vi "MGI Origin at Top Left.vi"(7 "Error In":errorcluster, 10 "VI Reference In (Caller)":refnum<vi>) -> (0 "Error Out":errorcluster, 3 "VI Reference Out":refnum<vi>)   [LabVIEW 2016]
doc: "Places the referenced VI's front panel's origin at the top left of the pane.\n\nAuthored by Robert C. Mortensen\nsupport@mooregoodideas.com\nwww.mooregoodideas.com\n\nCopyright (c) 2010, Moore Good Ideas, Inc.\n\nAll rights reserved.\n\nRedistribution and use in source and binary forms, with or without modification, are permitted provided that the following conditions are met:\n\n * Redistributions of source code must retain the above copyright notice, this list of conditions and the following disclaimer.\n * Redistributions in binary form must reproduce the above copyright notice, this list of conditions and the following disclaimer in the documentation and/or other materials provided with the distribution.\n * Neither the name of Moore Good Ideas, Inc. nor the names of its contributors may be used to endorse or promote products derived from this software without specific prior written permission.\n\nTHIS SOFTWARE IS PROVIDED BY THE COPYRIGHT HOLDERS AND CONTRIBUTORS \"AS IS\" AND ANY EXPRESS OR IMPLIED WARRANTIES, INCLUDING, BUT NOT LIMITED TO, THE IMPLIED WARRANTIES OF MERCHANTABILITY AND FITNESS FOR A PARTICULAR PURPOSE ARE DISCLAIMED. IN NO EVENT SHALL THE COPYRIGHT OWNER OR CONTRIBUTORS BE LIABLE FOR ANY DIRECT, INDIRECT, INCIDENTAL, SPECIAL, EXEMPLARY, OR CONSEQUENTIAL DAMAGES (INCLUDING, BUT NOT LIMITED TO, PROCUREMENT OF SUBSTITUTE GOODS OR SERVICES; LOSS OF USE, DATA, OR PROFITS; OR BUSINESS INTERRUPTION) HOWEVER CAUSED AND ON ANY THEORY OF LIABILITY, WHETHER IN CONTRACT, STRICT LIABILITY, OR TORT (INCLUDING NEGLIGENCE OR OTHERWISE) ARISING IN ANY WAY OUT OF THE USE OF THIS SOFTWARE, EVEN IF ADVISED OF THE POSSIBILITY OF SUCH DAMAGE."
uses:
  <vilib>/Utility/miscctls.llb/LVPointTypeDef.ctl
  <userlib>/_MGI/Application Control/MGI VI Reference/MGI Caller's VI Reference.vi
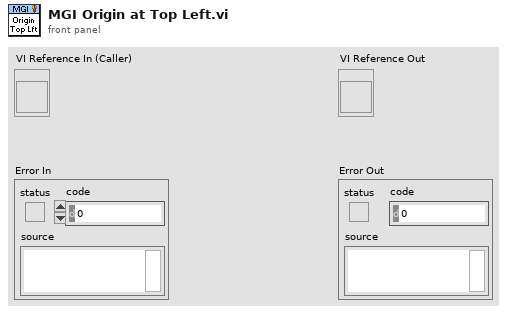
[diagram p1: front panel]
types:
  T1 = typedef "LVPointTypeDef.ctl" = cluster{"Horizontal":i16, "Vertical":i16}
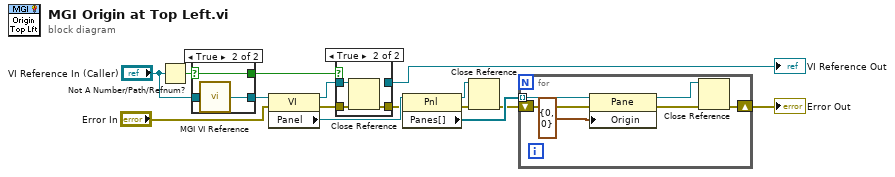
[diagram p0: block diagram]
diagram:
  n1 = Not A Number/Path/Refnum?(number/path/refnum="VI Reference In (Caller)") -> (NaN/Path/Refnum?=w6:bool)
  n2 = case shown="True" w6 {
    selector: w6 -> [_ w17]
    tunnel: [w16 w18] -> w4
    tunnel: "VI Reference In (Caller)" -> [w16 _]
    tunnel: [_ w17] -> w2
    frame False {
    }
    frame True {
      n3 = call-poly <userlib>:"MGI VI Reference.vi"() -> ("Caller's VI Reference"=w18:refnum<vi>)  [unwired: 1 in]
    }
  }
  n4 = property class="VI"(reference=w4, error in="Error In") -> (reference out=w12:refnum<vi>, error out=w13:errorcluster, "Panel"=w15:refnum<vi>)
  n5 = case shown="True" w2 {
    tunnel: w13 -> [w20 w23]
    tunnel: w12 -> [w19 w22]
    tunnel: [w20 w21] -> w11
    tunnel: [w19 _] -> w1
    frame False {
    }
    frame True {
      n6 = Close Reference(reference=w22, error in (no error)=w23) -> (error out=w21:errorcluster)
    }
  }
  "VI Reference Out" <- w1
  n7 = property class="Pnl"(reference=w15, error in=w11) -> (reference out=w8:refnum<vi>, error out=w9:errorcluster, "Panes[]"=w14:refnum<vi>[])
  n8 = Close Reference(reference=w8, error in (no error)=w9) -> (error out=w10:errorcluster)
  n9 = for {
    tunnel: w14 -> [w28] mode=indexing
    shift-right: [w25] -> w7
    shift-left: w10 -> [w29]
    n10 = property class="Pane"(reference=w28, error in=w29, "Origin"=T1 {"Horizontal"=0, "Vertical"=0} ("Horizontal Scrollbar Visibility")) -> (reference out=w26:refnum<vi>, error out=w27:errorcluster)
    n11 = Close Reference(reference=w26, error in (no error)=w27) -> (error out=w25:errorcluster)
  }
  "Error Out" <- w7
